vi "ReadChannel.vi"(8 "error in (no error)":errorcluster, 11 "I2C in":refnum<class "I2C.lvclass">) -> (0 "error out":errorcluster, 2 "I2C Channel":u8, 3 "I2C out":refnum<class "I2C.lvclass">)   [LabVIEW 2014, in "I2C.lvclass"]
doc: "Returns the I2C channel in use."
uses:
  I2C.lvclass
  I2C.lvclass/I2C.ctl
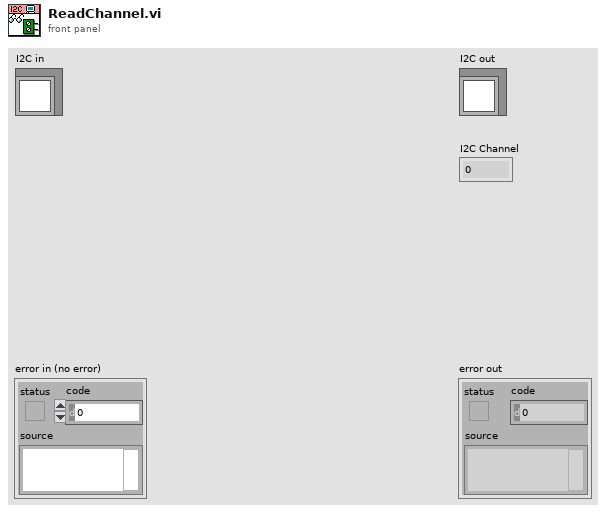
[diagram p1: front panel]
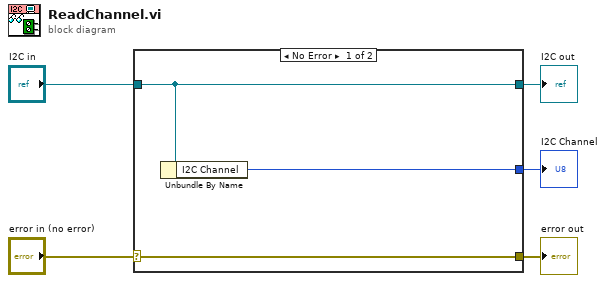
[diagram p0: block diagram]
diagram:
  n1 = case shown="No Error" "error in (no error)" {
    selector: "error in (no error)" -> [w8 w9]
    tunnel: [w8 w9] -> w4
    tunnel: [w7 w10] -> w2
    tunnel: "I2C in" -> [w7 w10]
    tunnel: [w6 _] -> w1
    frame No Error {
      n2 = Unbundle By Name(w7) -> ("I2C Channel"=w6:u8)
    }
    frame Error {
    }
  }
  "error out" <- w4
  "I2C out" <- w2
  "I2C Channel" <- w1
